vi "String into Number.vi"(1 "initial scan location":u32=4, 2 "String":string) -> (0 "output 1":i32)   [LabVIEW 2014]
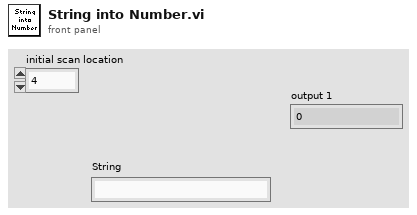
[diagram p1: front panel]
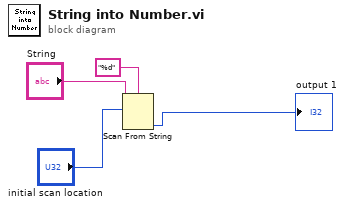
[diagram p0: block diagram]
diagram:
  n1 = Scan From String(format string="%d", input string="String", initial scan location="initial scan location") -> (output 1=→"output 1":i32)  [unwired: 2 in, 3 out]
